vi "Simple-Receiver.vi"() -> ()   [LabVIEW 2016]
panel:
  in  "Stop":bool
  out "Received Data":dbl(graph)
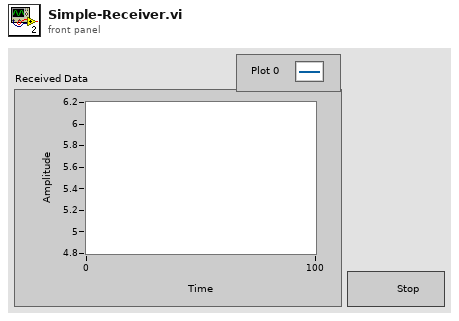
[diagram p1: front panel]
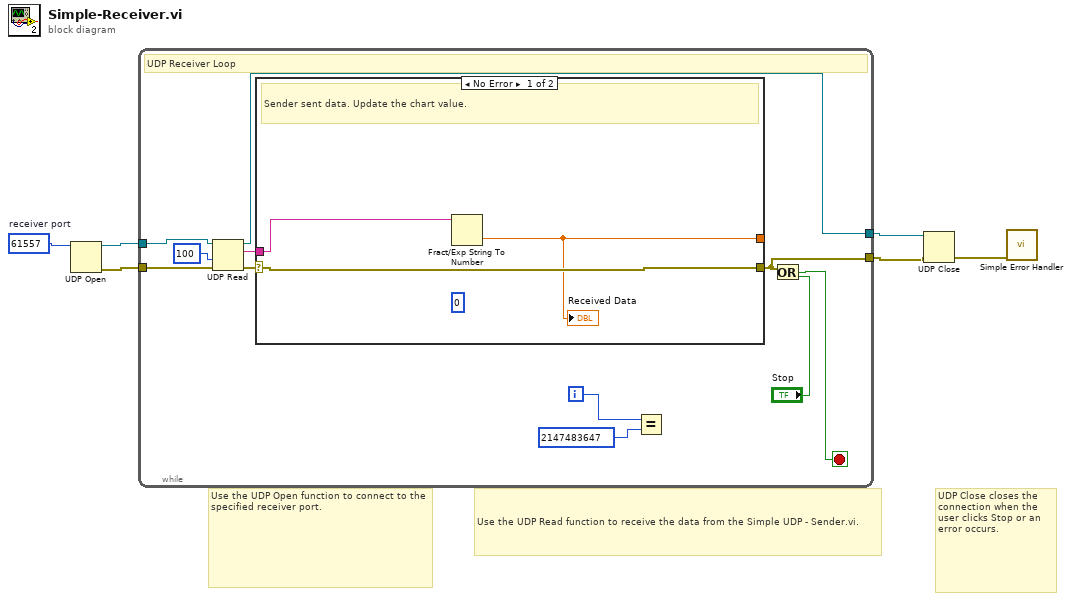
[diagram p0: block diagram]
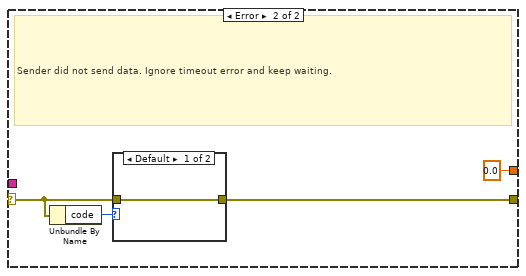
[diagram p2: hidden frame]
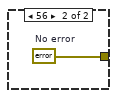
[diagram p3: hidden frame]
diagram:
  w1 = u16 61557  # receiver port
  # "UDP Close closes the connection when the user clicks Stop or an error occurs."
  # "Use the UDP Open function to connect to the specified receiver port."
  # "Use the UDP Read function to receive the data from the Simple UDP - Sender.vi."
  n1 = UDP Open(11:w1) -> (port=w2:refnum<k16>, 0:w3:errorcluster)  [unwired: 4 in, 1 out]
  n2 = while {
    tunnel: w2 -> [w17]
    tunnel: [w10] -> w6
    tunnel: w3 -> [w15]
    tunnel: [w11] -> w4
    i -> [w9]
    stop <- w7 stop-if-true
    # "UDP Receiver Loop"
    n3 = UDP Read(connection ID=w17, timeout ms (25000)=100, 8:w15) -> (data out=w13:string, error out=w12:errorcluster, 3:w10:refnum<k16>)  [unwired: 3 out]
    n4 = case shown="No Error" w12 {
      selector: w12 -> [w20 w23]
      tunnel: w13 -> [w19 _]
      tunnel: [w20 w22] -> w11
      tunnel: [w18 0.0] -> _
      frame No Error {
        (unwired) 0 ("offset (0)")
        # "Sender sent data. Update the chart value."
        n5 = Fract/Exp String To Number(string=w19) -> (number=w18:dbl)  [unwired: 3 in, 1 out]
        "Received Data" <- w18
      }
      frame Error {
        # "Sender did not send data. Ignore timeout error and keep waiting."
        n6 = Unbundle By Name(w23) -> ("code"=w24:i32)
        n7 = case shown="Default" w24 {
          tunnel: w23 -> [w25 _]
          tunnel: [w25 w26] -> w22
          frame Default {
          }
          frame 56 {
            w26 = errorcluster {"status"=FALSE, "code"=0, "source"=""}  # No error
          }
        }
      }
    }
    n8 = Equal?(x=w9, y=2147483647) -> ()  [unwired: 1 out]
    n9 = Or(x=w11, y="Stop") -> (x .or. y?=w7:bool)
  }
  n10 = UDP Close(connection ID=w6, 8:w4) -> (error out=w5:errorcluster)  [unwired: 1 out]
  n11 = call <vilib>:"Simple Error Handler.vi"("error in (no error)"=w5) -> ()  [unwired: 1 in, 8 out]
